vi "SystemsUI.vi"() -> ()   [LabVIEW 2013, in "PL Framework Configuration Tool.lvlib" / "Systems.lvclass"]
doc: "This VI is a template of the minimun components for a node UI.\nIt shows how to use the queue and the user event."
uses:
  Systems.lvclass
  <vilib>/NI/Configuration Framework/Node/NodeRef.ctl
  <vilib>/NI/Configuration Framework/Node/NISE_CEF_Node.lvclass
  <vilib>/NI/AMC/Message Queue.ctl
  <vilib>/NI/AMC/Message.ctl
  <vilib>/NI/Tools/Keyed Array/KeyedArray.ctl
  <vilib>/NI/Configuration Framework/Node/UserEventRef.ctl
  <vilib>/NI/Configuration Framework/Controls/EventCluster.ctl
  <vilib>/NI/Configuration Framework/Node/RefreshUIEvent.ctl
  <vilib>/NI/Configuration Framework/Node/CacheState.ctl
  <vilib>/NI/Configuration Framework/Node/StopEvent.ctl
  <vilib>/NI/Configuration Framework/Node/NodeChangeEvent.ctl
  <vilib>/Utility/miscctls.llb/LVPositionTypeDef.ctl
  Systems.lvclass/Systems.ctl
  Framework Configuration Classes/system configuration/PL_System Configuration.lvclass/PL_System Configuration.ctl
  <vilib>/NI/Configuration Framework/serializable configuration/set alias.vi
  <vilib>/NI/Configuration Framework/serializable configuration/get alias.vi
  Framework Configuration Classes/system configuration/PL_System Configuration.lvclass
  <vilib>/National Instruments/DCAF UI Toolkit/Controls/DCAF UI Elements.lvlib
  <vilib>/NI/Tools/Keyed Array/Tools_KeyedArray.lvlib
  <vilib>/NI/AMC/AMC.lvlib
  <vilib>/NI/Configuration Framework/NISE_CEF_TreeControl.lvlib
panel:
  in  "Top Level Tab Control":enum32{"Configuration Settings"}(tab)
  in  "Configuration Name":string
  in  "Major":u8=1 min=1
  in  "Minor":u8
  in  "Fix":u8
  in  "Build":u8=1 min=1
  in  "Description":string
  out "Time Last Saved 2":string
  in  "node change":T1
  in  "stop event":T2
  in  "cache state":T3
  in  "refresh UI":T4
  in  "user event":T5
  in  "main queue":T6
  in  "node ref":T7
  # "Revision"
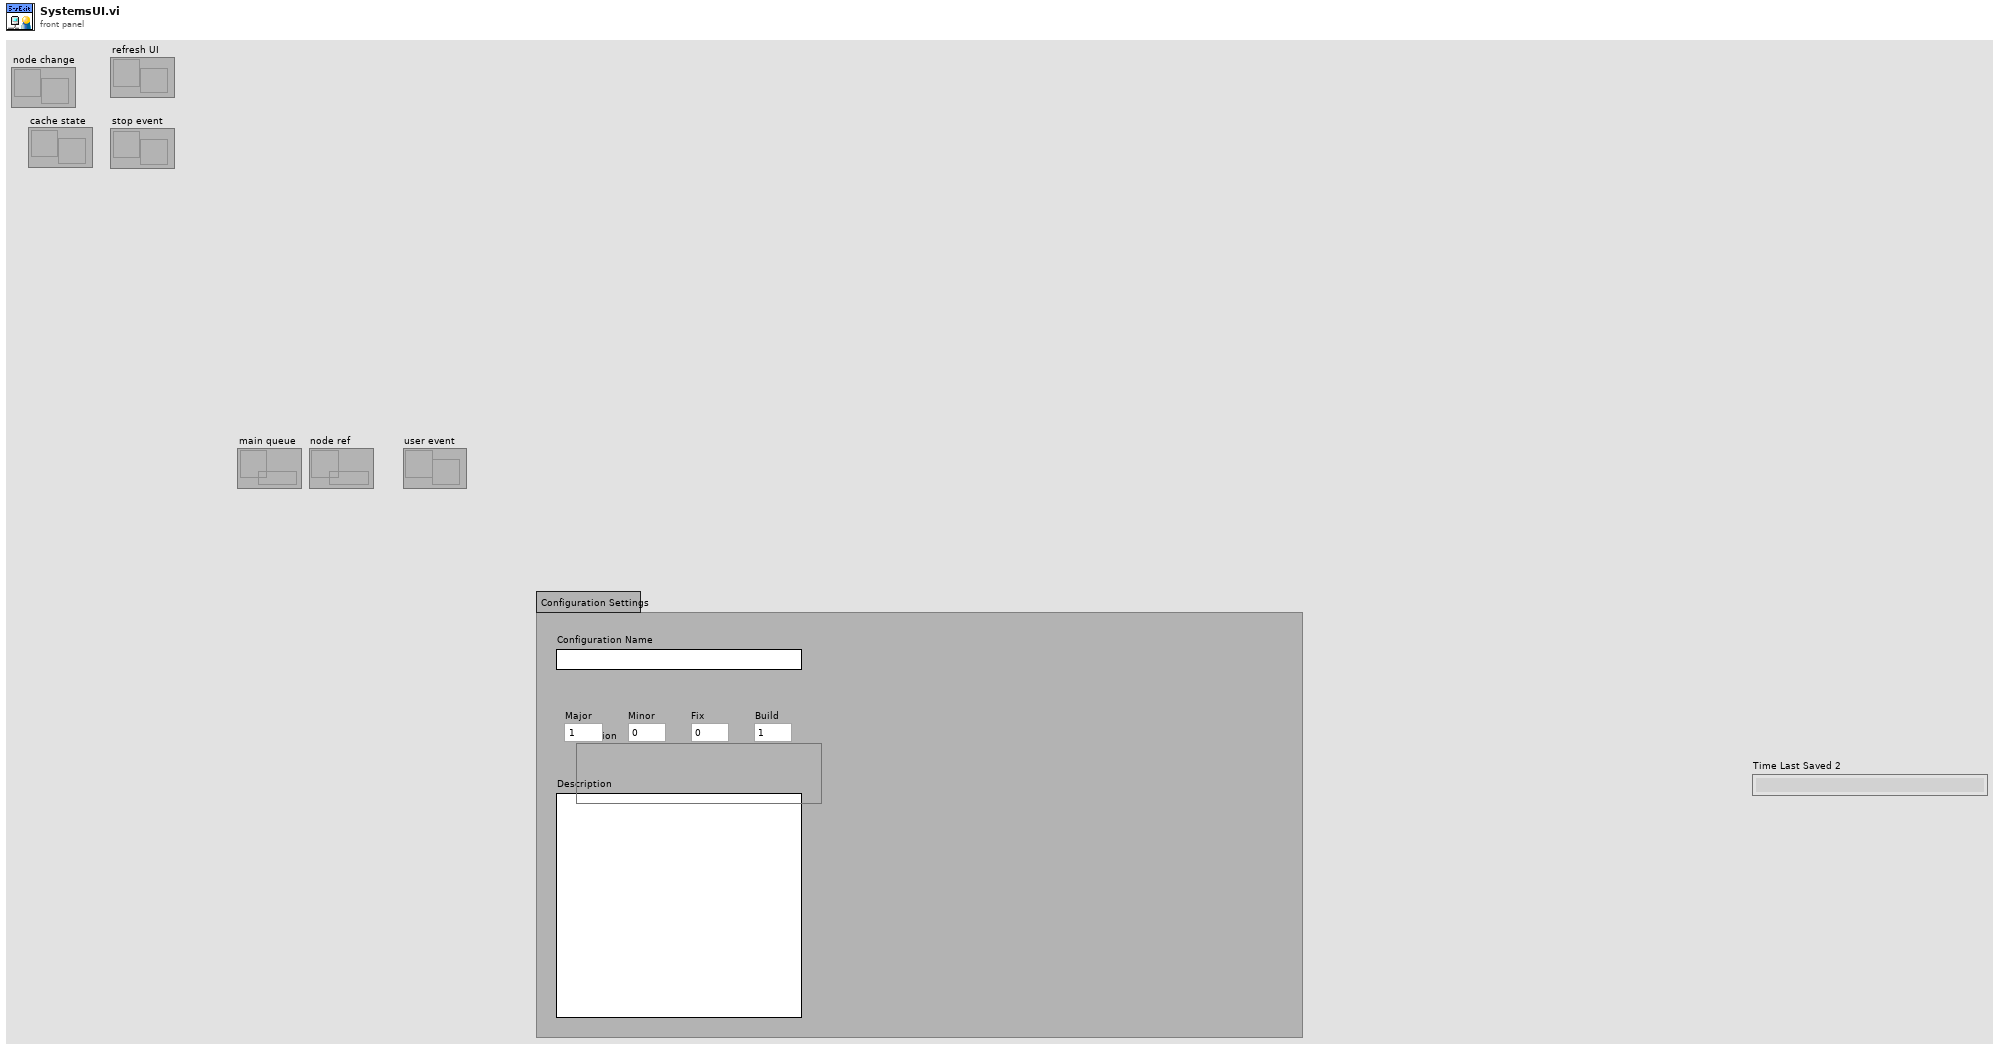
[diagram p1: front panel]
types:
  T1 = typedef "NISE_CEF_Node.lvclass/NodeChangeEvent.ctl" = refnum<user-event>
  T2 = typedef "NISE_CEF_Node.lvclass/StopEvent.ctl" = refnum<user-event>
  T3 = typedef "NISE_CEF_Node.lvclass/CacheState.ctl" = refnum<user-event>
  T4 = typedef "NISE_CEF_Node.lvclass/RefreshUIEvent.ctl" = refnum<user-event>
  T5 = typedef "NISE_CEF_Node.lvclass/UserEventRef.ctl" = refnum<user-event>
  T6 = typedef "AMC.lvlib/Message Queue.ctl" = refnum<queue>
  T7 = typedef "NISE_CEF_Node.lvclass/NodeRef.ctl" = refnum<data-value>
  T8 = typedef "LVPositionTypeDef.ctl" = cluster{"Left":i32, "Top":i32}
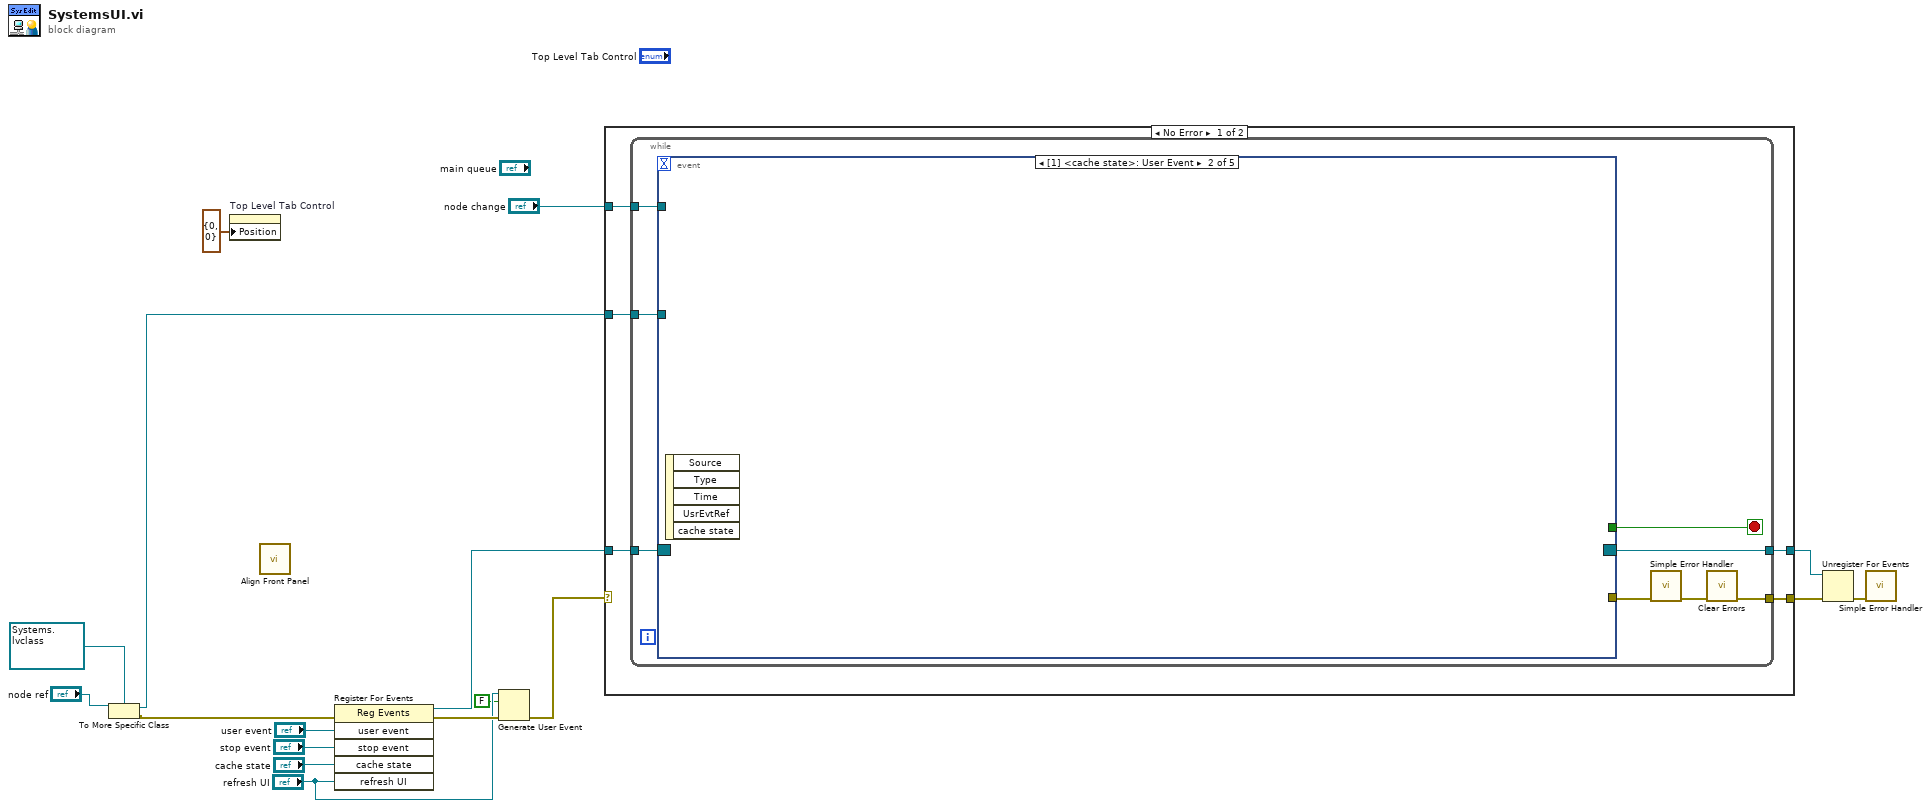
[diagram p0: block diagram]
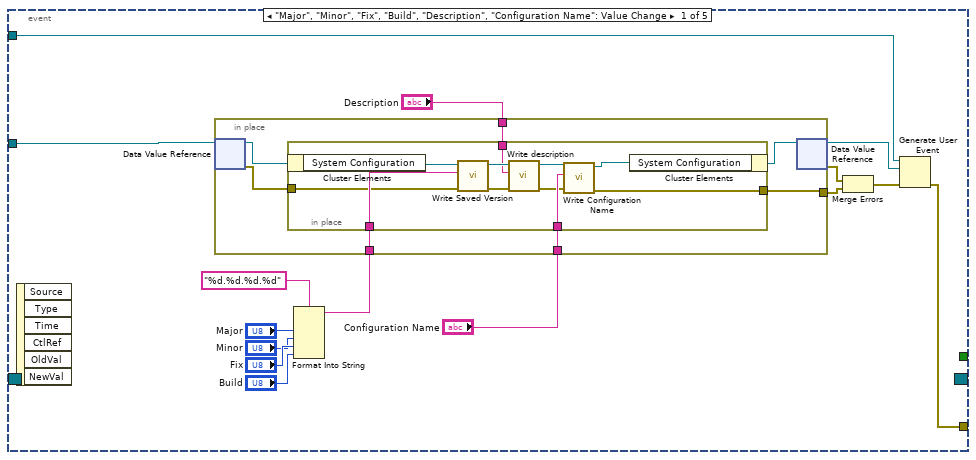
[diagram p2: hidden frame]
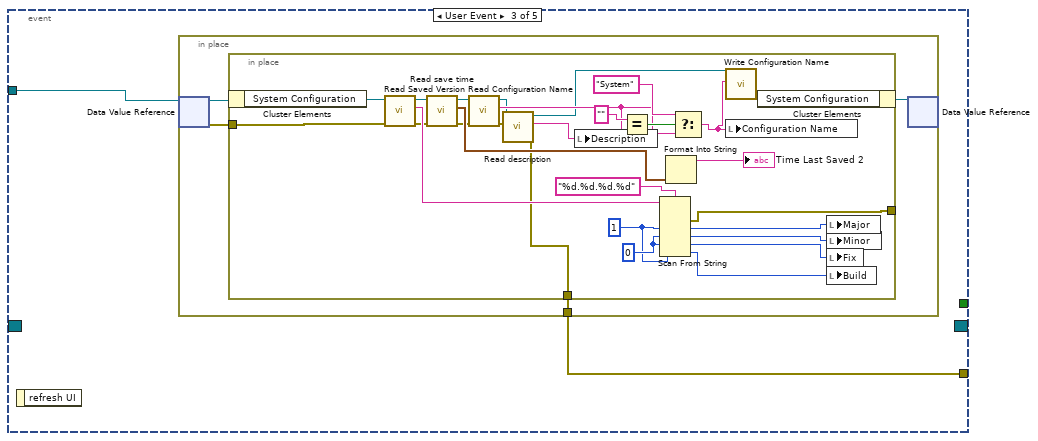
[diagram p3: hidden frame]
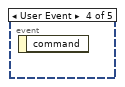
[diagram p4: hidden frame]
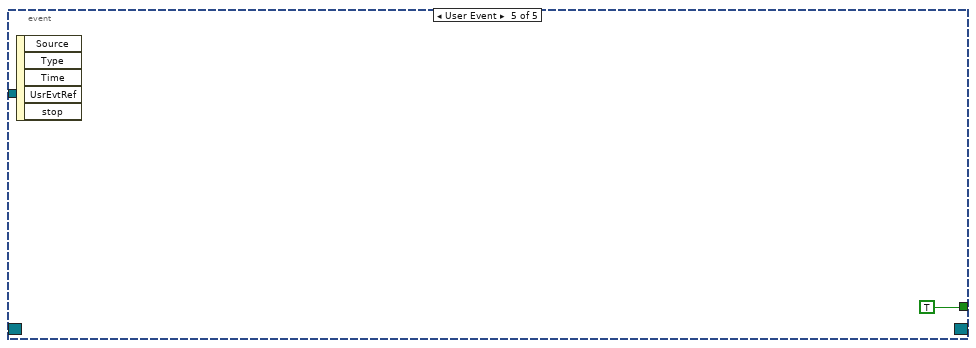
[diagram p5: hidden frame]
diagram:
  n1 = To More Specific Class(target class=refnum<data-value> refnum ("data value reference"), reference="node ref") -> (specific class reference=w2:refnum<data-value>, error out=w3:errorcluster)  [unwired: 1 in]
  n2 = property on="Top Level Tab Control" class="TabCtl (strict)"("Position"=T8 {"Left"=0, "Top"=0}) -> ()  [unwired: 2 in, 2 out]
  n3 = call <vilib>:"Align Front Panel.vi"() -> ()  [unwired: 10 in, 2 out]
  n4 = register-events(error in=w3, "user event", "stop event", "cache state", "refresh UI") -> (reference out=w16:refnum<event-registration>, error out=w13:errorcluster)  [unwired: 1 in]
  n5 = Generate User Event(user event="refresh UI", event data cluster=FALSE ("event data"), error in=w13) -> (error out=w5:errorcluster)  [unwired: 1 in, 1 out]
  n6 = case shown="No Error" w5 {
    selector: w5 -> [_ w100]
    tunnel: w2 -> [w22 _]
    tunnel: w16 -> [w21 w99]
    tunnel: [w20 w99] -> w15
    tunnel: [w19 w100] -> w14
    tunnel: "node change" -> [w18 _]
    frame No Error {
      n7 = while {
        tunnel: w22 -> [w30]
        tunnel: w21 -> [w29]
        tunnel: [w28] -> w20
        tunnel: [w23] -> w19
        tunnel: w18 -> [w25]
        stop <- w27 stop-if-true
        n8 = event shown="[1] <cache state>: User Event" {
          selector: w29 -> [_ _ _ _ _]
          dyn-events: [_ _ _ _ _] -> w28
          timeout: _ -> [_ _ _ _ _]
          tunnel: w30 -> [w45 _ w64 _ _]
          tunnel: [_ _ _ _ TRUE] -> w27
          tunnel: [w31 _ w65 _ _] -> w26
          tunnel: w25 -> [w33 _ _ _ _]
          event "Major", "Minor", "Fix", "Build", "Description", "Configuration Name": Value Change {
            n9 = event-data() -> ()  [unwired: 1 in, 6 out]
            n10 = Format Into String(format string="%d.%d.%d.%d", "Major", "Minor", "Fix", "Build") -> (resulting string=w38:string)  [unwired: 2 in, 1 out]
            n11 = in-place {
              in-place-border: "Description" -> [w50]
              in-place-border: w38 -> [w49]
              in-place-border: "Configuration Name" -> [w48]
              in-place-border: [w46] -> w36
              n12 = in-place-dvr #1(w45) -> (w52:refnum<class "Systems.lvclass">, w47:errorcluster)
              n13 = in-place {
                in-place-border: w49 -> [w61]
                in-place-border: w50 -> [w60]
                in-place-border: w48 -> [w57]
                in-place-border: w47 -> [w56]
                in-place-border: [w53] -> w46
                n14 = in-place-cluster #2(w52) -> ("System Configuration"=w63:refnum<class "PL_System Configuration.lvclass">)
                n15 = call "Write Saved Version.vi"("error in"=w56, "Saved Version"=w61, "PL_System Configuration in"=w63) -> ("error out"=w55:errorcluster, "PL_System Configuration out"=w62:refnum<class "PL_System Configuration.lvclass">)  [unwired: 7 in]
                n16 = call "Write description.vi"("error in"=w55, "description"=w60, "PL_System Configuration in"=w62) -> ("error out"=w54:errorcluster, "PL_System Configuration out"=w59:refnum<class "PL_System Configuration.lvclass">)  [unwired: 7 in]
                n17 = call "Write Configuration Name.vi"("error in"=w54, "Configuration Name"=w57, "PL_System Configuration in"=w59) -> ("error out"=w53:errorcluster, "PL_System Configuration out"=w58:refnum<class "PL_System Configuration.lvclass">)  [unwired: 7 in]
                n18 = in-place-cluster #2("System Configuration"=w58) -> (w51:refnum<class "Systems.lvclass">)
              }
              n19 = in-place-dvr #1(w51) -> (w32:refnum<data-value>, w35:errorcluster)
            }
            n20 = Merge Errors(w35, w36) -> (w34:errorcluster)
            n21 = Generate User Event(user event=w33, event data cluster=w32, error in=w34) -> (error out=w31:errorcluster)  [unwired: 1 in, 1 out]
          }
          event User Event {
            n22 = event-data() -> ()  [unwired: 1 in, 5 out]
          }
          event User Event {
            n23 = event-data() -> ()  [unwired: 1 in, 1 out]
            n24 = in-place {
              in-place-border: [w66] -> w65
              n25 = in-place-dvr #3(w64) -> (w69:refnum<class "Systems.lvclass">, w67:errorcluster)
              n26 = in-place {
                in-place-border: w67 -> [w78]
                in-place-border: [w75] -> w66
                in-place-border: [w87] -> _
                w93 = u8 0
                w92 = u8 1
                n27 = in-place-cluster #4(w69) -> ("System Configuration"=w79:refnum<class "PL_System Configuration.lvclass">)
                n28 = call "Read Saved Version.vi"("error in"=w78, "PL_System Configuration in"=w79) -> ("error out"=w77:errorcluster, "Saved Version"=w83:string, "PL_System Configuration out"=w80:refnum<class "PL_System Configuration.lvclass">)  [unwired: 7 in]
                n29 = call "Read save time.vi"("error in"=w77, "PL_System Configuration in"=w80) -> ("error out"=w76:errorcluster, "save time"=w84:timestamp, "PL_System Configuration out"=w81:refnum<class "PL_System Configuration.lvclass">)  [unwired: 7 in]
                n30 = call "Read Configuration Name.vi"("error in"=w76, "PL_System Configuration in"=w81) -> ("error out"=w82:errorcluster, "Configuration Name"=w85:string, "PL_System Configuration out"=w74:refnum<class "PL_System Configuration.lvclass">)  [unwired: 7 in]
                n31 = call "Read description.vi"("error in"=w82, "PL_System Configuration in"=w74) -> ("error out"=w75:errorcluster, "description"=w72:string, "PL_System Configuration out"=w73:refnum<class "PL_System Configuration.lvclass">)  [unwired: 7 in]
                n32 = local write "Description"(w72) -> ()
                n33 = Equal?(x="" ("y"), y=w85) -> (x = y?=w97:bool)
                n34 = Scan From String(format string="%d.%d.%d.%d", input string=w83, default 1=w92, default 2=w93, default 3=w93, default 4=w92) -> (error out=w87:errorcluster, output 1=w88:u8, output 2=w89:u8, output 3=w90:u8, output 4=w91:u8)  [unwired: 2 in, 2 out]
                n35 = Format Into String(w84) -> (resulting string=→"Time Last Saved 2":string)  [unwired: 3 in, 1 out]
                n36 = Select(t="System", s=w97, f=w85) -> (s? t:f=w70:string)
                n37 = call "Write Configuration Name.vi"("Configuration Name"=w70, "PL_System Configuration in"=w73) -> ("PL_System Configuration out"=w71:refnum<class "PL_System Configuration.lvclass">)  [unwired: 8 in, 1 out]
                n38 = local write "Configuration Name"(w70) -> ()
                n39 = in-place-cluster #4("System Configuration"=w71) -> (w68:refnum<class "Systems.lvclass">)
                n40 = local write "Major"(w88) -> ()
                n41 = local write "Minor"(w89) -> ()
                n42 = local write "Fix"(w90) -> ()
                n43 = local write "Build"(w91) -> ()
              }
              n44 = in-place-dvr #3(w68) -> ()  [unwired: 2 out]
            }
          }
          event User Event {
            n45 = event-data() -> ()  [unwired: 1 in, 1 out]
          }
          event User Event {
            n46 = event-data() -> ()  [unwired: 1 in, 5 out]
          }
        }
        n47 = call <vilib>:"Simple Error Handler.vi"("error in (no error)"=w26) -> ("error out"=w24:errorcluster)  [unwired: 4 in, 4 out]
        n48 = call <vilib>:"Clear Errors.vi"("error in (no error)"=w24) -> ("error out"=w23:errorcluster)  [unwired: 6 in]
      }
    }
    frame Error {
    }
  }
  n49 = Unregister For Events(event registration refnum=w15, error in=w14) -> (error out=w4:errorcluster)
  n50 = call <vilib>:"Simple Error Handler.vi"("error in (no error)"=w4) -> ()  [unwired: 4 in, 5 out]
